vi "Read All Namespaces.vi"(8 "error in (no error)":errorcluster, 11 "TwinCAT ADS in":refnum<class "TwinCAT ADS.lvclass">) -> (0 "error out":errorcluster, 2 "Namespaces":string[](array[string]), 3 "TwinCAT ADS out":refnum<class "TwinCAT ADS.lvclass">)   [LabVIEW 2018, in "TwinCAT ADS.lvclass"]
uses:
  TwinCAT ADS.lvclass
  TwinCAT ADS.lvclass/TwinCAT ADS.ctl
  TwinCAT.Ads
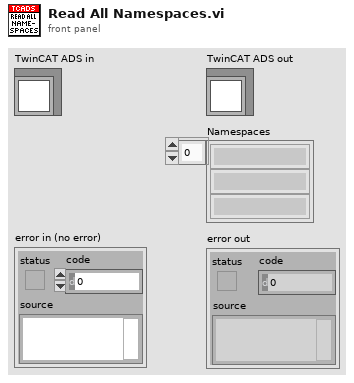
[diagram p1: front panel]
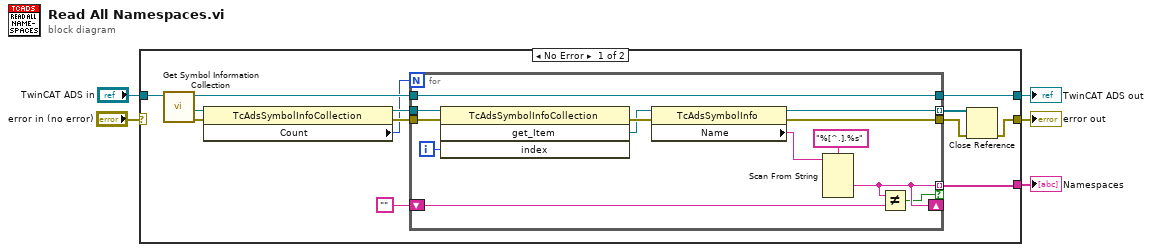
[diagram p0: block diagram]
diagram:
  n1 = case shown="No Error" "error in (no error)" {
    selector: "error in (no error)" -> [_ w33]
    tunnel: [w11 w33] -> w4
    tunnel: [w15 w32] -> w2
    tunnel: "TwinCAT ADS in" -> [w18 w32]
    tunnel: [w13 _] -> w1
    frame No Error {
      n2 = call "Get Symbol Information Collection.vi"("TwinCAT ADS in"=w18) -> ("error out"=w10:errorcluster, ".NET AdsSymbolInfoCollection"=w9:refnum<k24>, "TwinCAT ADS out"=w17:refnum<class "TwinCAT ADS.lvclass">)  [unwired: 8 in]
      n3 = property class="TcAdsSymbolInfoCollection"(reference=w9, error in=w10) -> (reference out=w7:refnum<k24>, error out=w8:errorcluster, "Count"=w6:i32)
      n4 = for {
        N: w6 -> [_]
        tunnel: w17 -> [w31]
        tunnel: w8 -> [w23]
        tunnel: [w31] -> w15
        tunnel: [w30] -> w16 mode=indexing
        tunnel: [w29] -> w12
        tunnel: [w26] -> w13 mode=indexing if=w25
        shift-right: [w26] -> _
        shift-left: "" -> [w24]
        tunnel: w7 -> [w21]
        i -> [w22]
        n5 = invoke class="TcAdsSymbolInfoCollection" method="get_Item"(reference=w21, error in=w23, "index"=w22) -> (error out=w20:errorcluster, "get_Item"=w19:refnum<k24>)  [unwired: 1 in, 2 out]
        n6 = property class="TcAdsSymbolInfo"(reference=w19, error in=w20) -> (reference out=w30:refnum<k24>, error out=w29:errorcluster, "Name"=w27:string)
        n7 = Scan From String(format string="%[^.].%s", input string=w27) -> (output 1=w26:string)  [unwired: 5 in, 3 out]
        n8 = Not Equal?(x=w26, y=w24) -> (x != y?=w25:bool)
      }
      n9 = Close Reference(reference=w16, error in (no error)=w12) -> (error out=w11:errorcluster)
    }
    frame Error {
    }
  }
  "error out" <- w4
  "TwinCAT ADS out" <- w2
  "Namespaces" <- w1
